vi "RT_PCC_Control_v02b_clean.vi"() -> ()   [LabVIEW 2015]
uses:
  subVIs/PCC case typedef.ctl
  subVIs/Data_Queue_Command.ctl
  <vilib>/Platform/TimedLoop/XDataNode/timing_clust.ctl
  <vilib>/Platform/TimedLoop/XDataNode/nitl_modes.ctl
  <vilib>/Platform/TimedLoop/XDataNode/wakeup.ctl
  <vilib>/FPGAPlugInAG/cRIO-9068/niLvFpga_Open_cRIO-9068.vi
  <vilib>/rvi/interface/common/dynamic/niFpgaDynamicAddResources.vi
  <vilib>/Utility/error.llb/Error Cluster From Error Code.vi
  <vilib>/rvi/errors/niLvFpgaAdjustHostInterfaceError.vi
  <vilib>/FPGAPlugInAG/Dynamic/niLvFpga_Close_Dynamic.vi
  <vilib>/Modbus/slave/Create Slave Instance (TCP).vi
  <vilib>/Platform/TimedLoop/XDataNode/XDataNode.xnode
  <vilib>/rvi/interface/nirviOpenFPGA/nirviOpenFPGA.xnode
  FPGA Bitfiles/RTDSPCCControl_FPGA_RTDS_PCC_v02b_clean.lvbitx
  <vilib>/rvi/interface/nirviReadWriteControl/nirviReadWriteControl.xnode
  <vilib>/rvi/interface/nirviCloseFPGA/nirviCloseFPGA.xnode
  <vilib>/Modbus/slave/Modbus Slave.lvclass
  NiFpgaLv.dll
  <vilib>/rvi/interface/Simulation/niFpgaSimulationCallBeginRW.vi
  2015 SP1 Support Files/Project Dependencies/Common/Modbus Data Conversion.llb/Modbus Data Conversion.lvlib
  <vilib>/Platform/TimedLoop/XDataNode/XDNodeRunTimeDep.lvlib
panel:
  out "Paused?":bool
  in  "unpause":bool
  out "Enable Resync":bool
  out "Graph Data":sgl[][](graph)
  out "state machine loop time":u32
  out "PLL Time MG":u32
  in  "RMS reset":bool
  out "Grid Voltage":sgl[][](graph)
  out "Current":sgl[][](graph)
  out "Grid Freq":sgl[][](graph)
  in  "LPF enable":bool=TRUE
  out "RMS Time":u32
  out "Resync Time":u32
  out "S, P, & Q":cluster{sgl, sgl, sgl}(graph)
  in  "Use Angle for Q":bool
  out "error out":errorcluster
  out "RMS Computation Valid":bool
  out "Comm\nTimeout":bool
  out "V&I Cluster":cluster{sgl, sgl, sgl, sgl, sgl, sgl}
  out "P Cluster":cluster{sgl, sgl, sgl}
  out "S Cluster":cluster{sgl, sgl, sgl}
  out "Q Cluster":cluster{sgl, sgl, sgl}
  out "Q Total":sgl
  out "P Total":sgl
  out "S Total":sgl
  in  "Pause":bool
  out "Modbus Values":T1
  out "comm\nstopped":bool
  in  "Input Cluster":T1
  in  "Enable Switching":bool=TRUE
  out "Current state":T2
  in  "stop":bool
  out "Loop rate":u32=1332
  in  "Reset PLL":bool
  out "Open Switch":bool
  out "Close Switch":bool
  out "Switch Closed?":bool
  out "Activate Command":bool
  out "Deactivate Command":bool
  out "Activation Status":bool
  out "Deactivation Status":bool=TRUE
  out "TCP \nConnection Count":u32
  in  "Input register\naddresses":T3={"Ia RMS"=30030, "Ib RMS"=30040, "Ic RMS"=30050, "Vab RMS"=30130, "Vbc RMS"=30140, "Vca RMS"=30150, "Pa"=30230, "Pb"=30240, "Pc"=30250, "Qa"=30330, "Qb"=30340, "Qc"=30350}
  in  "Tab Control":enum32{"Resynchronization", "Normal Operation"}(tab)
  out "V RMS Resync":cluster{dbl, dbl}(graph)
  out "Freq Resync":cluster{dbl, dbl}(graph)
  out "Phase Resync":cluster{dbl, dbl, dbl, dbl}(graph)
  out "V rms":cluster{sgl, sgl}(graph)
  # "IF Error 1 < Limit 1\nOR \n(Error 2 > Limit 2 AND Error 2 < Limit 1)\nTHEN\nResync"
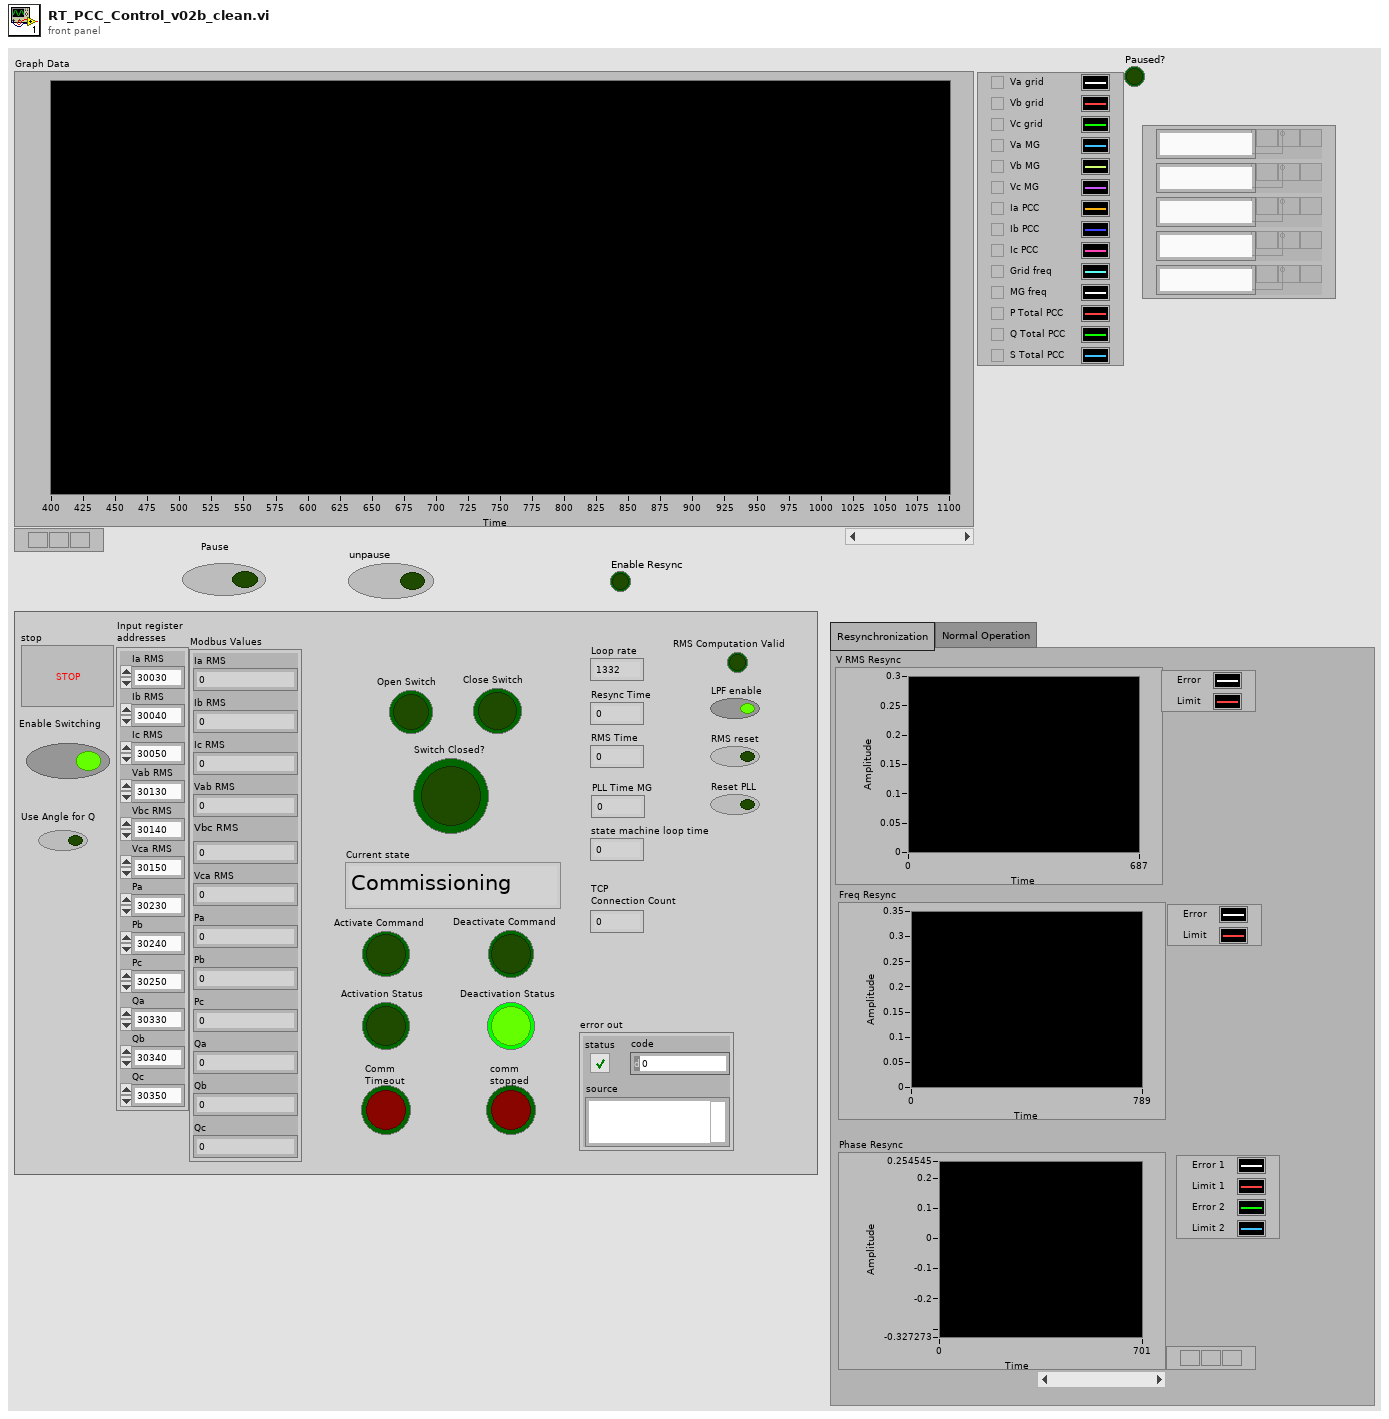
[diagram p1: front panel]
types:
  T1 = cluster{"Ia RMS":sgl, "Ib RMS":sgl, "Ic RMS":sgl, "Vab RMS":sgl, "Vbc RMS":sgl, "Vca RMS":sgl, "Pa":sgl, "Pb":sgl, "Pc":sgl, "Qa":sgl, "Qb":sgl, "Qc":sgl}
  T2 = typedef "PCC case typedef.ctl" = enum16{"Commissioning", "Open", "Synchronize check", "Synchronize", "Closed", "Island watch"}
  T3 = cluster{"Ia RMS":u16, "Ib RMS":u16, "Ic RMS":u16, "Vab RMS":u16, "Vbc RMS":u16, "Vca RMS":u16, "Pa":u16, "Pb":u16, "Pc":u16, "Qa":u16, "Qb":u16, "Qc":u16}
  T4 = typedef "Data_Queue_Command.ctl" = enum16{"Initialize", "Write Sample", "Pull Array", "Close"}
  T5 = typedef "XDNodeRunTimeDep.lvlib/timing_clust.ctl" = cluster{"Expected End [f-1]":u64, "Actual End [f-1]":u64, "Finished Late? [f-1]":bool, "Expected End [i-1]":u64, "Actual End [i-1]":u64, "Finished Late? [i-1]":bool, "Expected Start [i]":u64, "Actual Start [i]":u64, "Expected Start [f]":u64, "Actual Start [f]":u64, "Source Name":string, "Structure Name":string, "Period":i64, "Deadline":i64, "Offset":i64, "Start":i64, "Priority":i32, "Timeout":i32, "Mode":T6, "Wakeup Reason":T7, "Error":errorcluster, "Source Type":string, "Secondary Source Type":string, "Global End Time":u64, "Global Start Time":u64, "Frame Duration":u64, "Iteration Duration":u64, "Assigned CPU":i32, "I/O Scan Engine Mode":u32}
  T6 = typedef "XDNodeRunTimeDep.lvlib/nitl_modes.ctl" = enum32{"No Change", "Process missed periods, maintain original phase", "Discard missed periods, maintain original phase", "Process missed periods, ignore original phase", "Discard missed periods, ignore original phase"}
  T7 = typedef "XDNodeRunTimeDep.lvlib/wakeup.ctl" = enum32{"Normal", "Aborted", "Asynchronous wakeup", "Timing source error", "Timed loop error", "Timeout"}
  T8 = cluster{"Qa":fxp<+/-,46,10>, "Qb":fxp<+/-,46,10>, "Qc":fxp<+/-,46,10>}
  T9 = cluster{"Pa":fxp<+/-,32,10>, "Pb":fxp<+/-,32,10>, "Pc":fxp<+/-,32,10>}
  T10 = cluster{"Vab grid RMS":fxp<+,16,5>, "Vbc grid RMS":fxp<+,16,5>, "Vca grid RMS":fxp<+,16,5>, "Ia RMS":fxp<+,16,5>, "Ib RMS":fxp<+,16,5>, "Ic RMS":fxp<+,16,5>}
  T11 = cluster{"Vab grid RMS":sgl, "Vbc grid RMS":sgl, "Vca grid RMS":sgl, "Ia RMS":sgl, "Ib RMS":sgl, "Ic RMS":sgl}
  T12 = cluster{"Ia":fxp<+/-,24,5>, "Ib":fxp<+/-,24,5>, "Ic":fxp<+/-,24,5>}
  T13 = cluster{"Va":fxp<+/-,18,4>, "Vb":fxp<+/-,18,4>, "Vc":fxp<+/-,18,4>}
  T14 = cluster{"Va grid":sgl, "Vb grid":sgl, "Vc grid":sgl, "Ia":sgl, "Ib":sgl, "Ic":sgl}
  T15 = cluster{"Ia RMS":fxp<+,16,5>, "Ib RMS":fxp<+,16,5>, "Ic RMS":fxp<+,16,5>, "Vab grid RMS":fxp<+,16,5>, "Vbc grid RMS":fxp<+,16,5>, "Vca grid RMS":fxp<+,16,5>}
  T16 = cluster{"Ia RMS":sgl, "Ib RMS":sgl, "Ic RMS":sgl, "Vab grid RMS":sgl, "Vbc grid RMS":sgl, "Vca grid RMS":sgl}
  T17 = cluster{"Freq error":fxp<+,32,8>, "Freq constant":fxp<+,32,8>}
  T18 = cluster{"Phase angle error":fxp<+,32,1>, "Phase angle constant":fxp<+,32,1>, fxp<+/-,33,2>, "y":fxp<+,32,1>}
  T19 = cluster{fxp<+,27,5>, "Vgrid RMS constant (off grid)":fxp<+,27,5>}
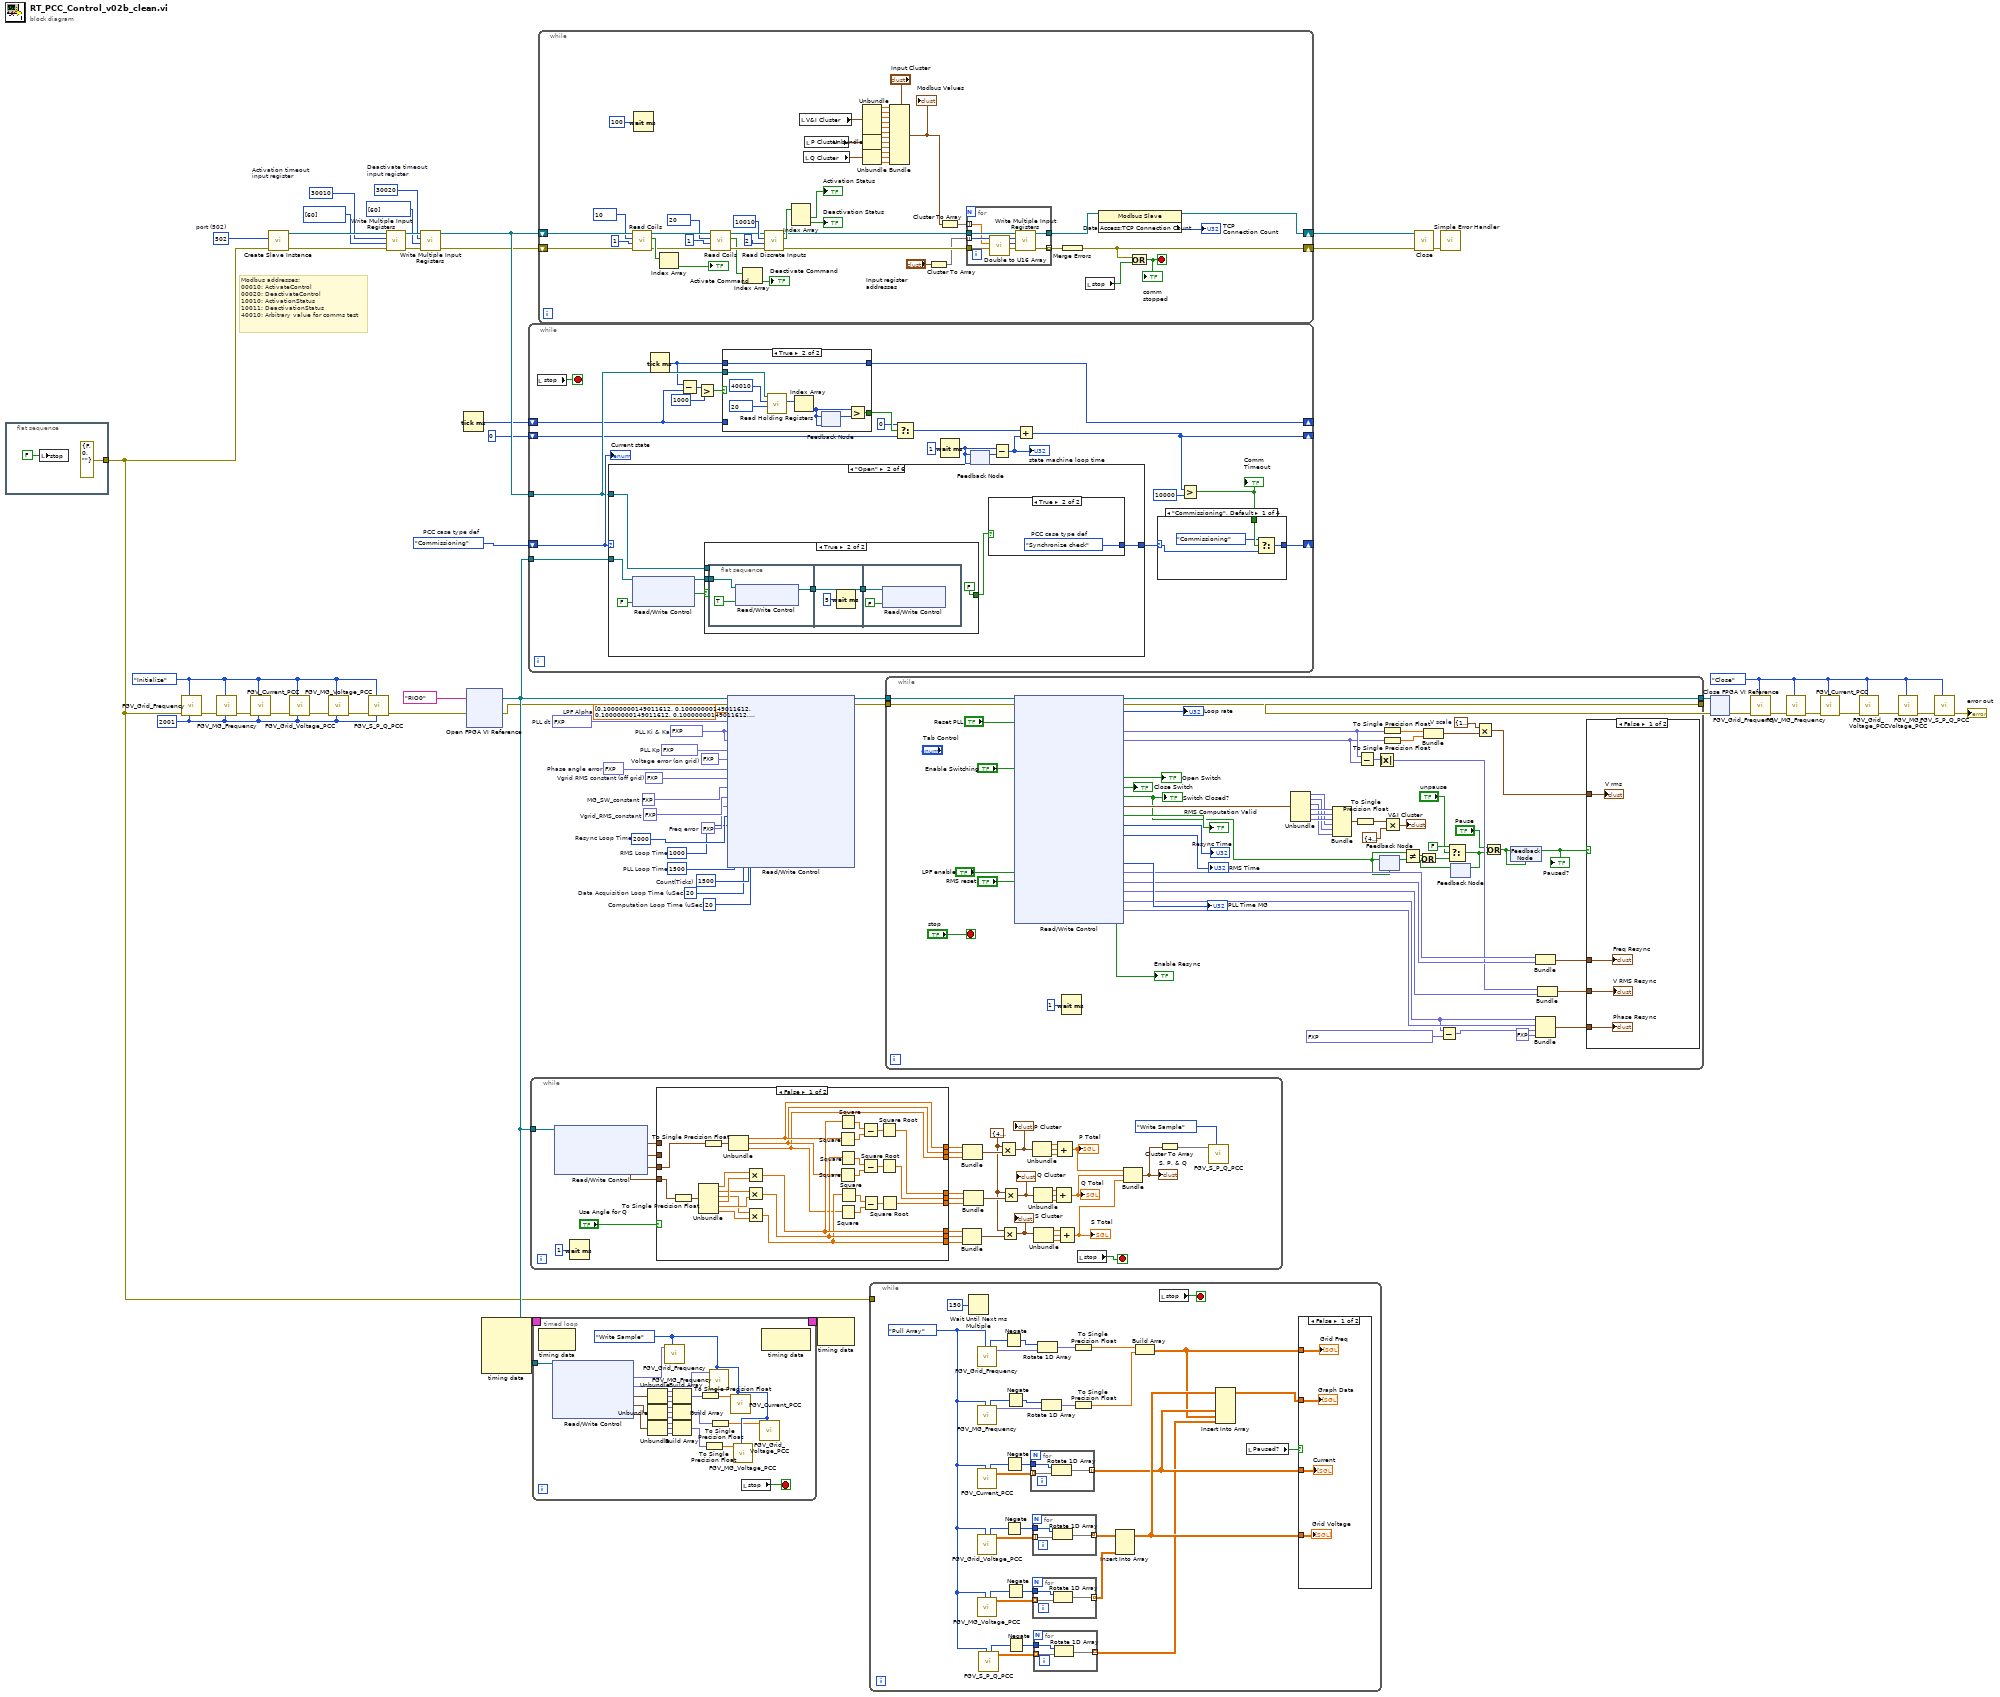
[diagram p0: block diagram]
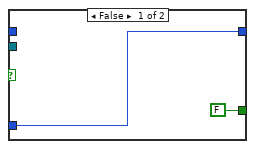
[diagram p2: hidden frame]
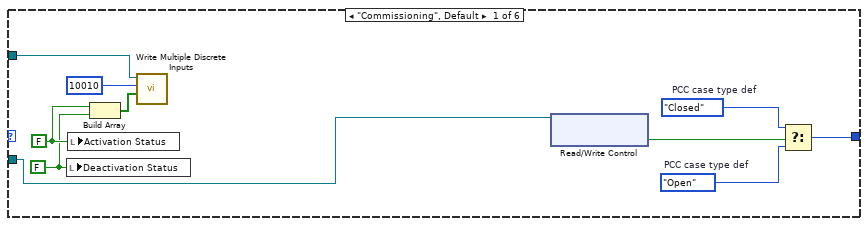
[diagram p6: hidden frame]
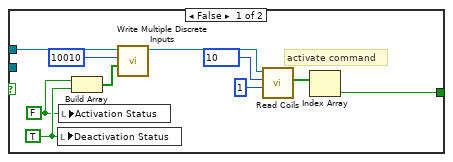
[diagram p7: hidden frame]
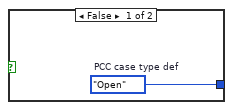
[diagram p8: hidden frame]
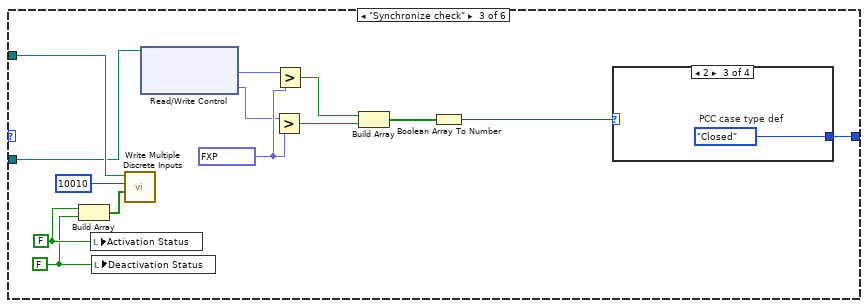
[diagram p9: hidden frame]
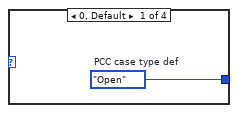
[diagram p10: hidden frame]
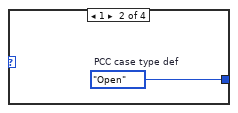
[diagram p11: hidden frame]
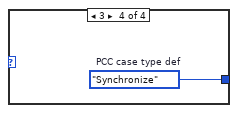
[diagram p12: hidden frame]
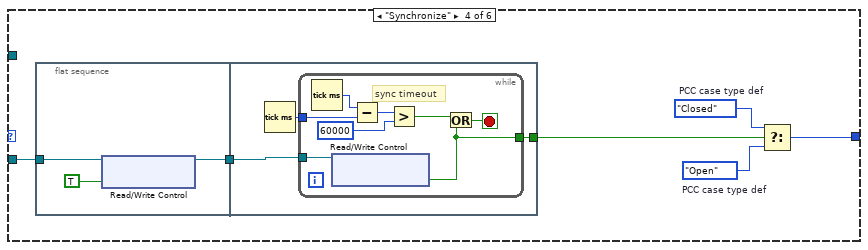
[diagram p13: hidden frame]
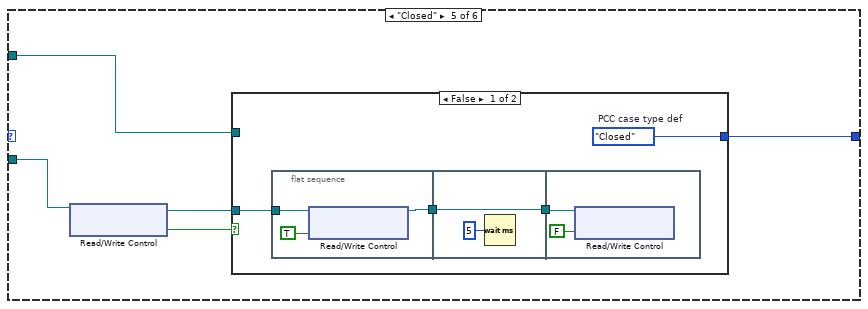
[diagram p14: hidden frame]
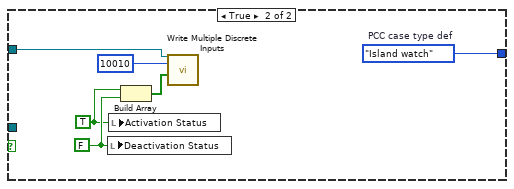
[diagram p15: hidden frame]
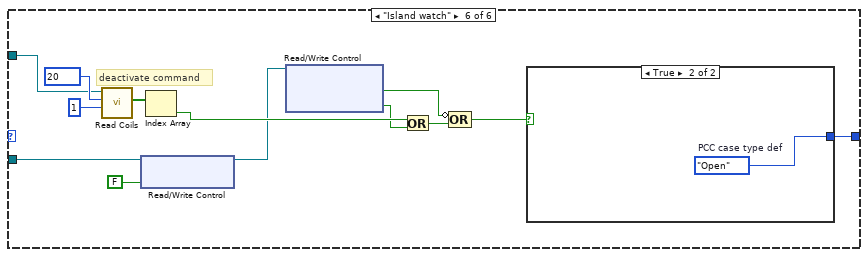
[diagram p16: hidden frame]
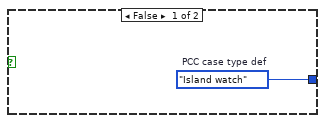
[diagram p17: hidden frame]
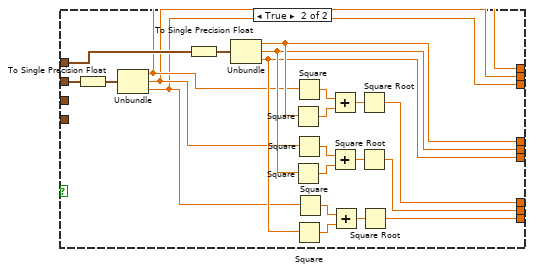
[diagram p19: hidden frame]
diagram:
  w56 = u16 502  # port (502)
  w9 = u32 20  # Computation Loop Time (uSec)
  w10 = u32 20  # Data Acquisition Loop Time (uSec)
  w11 = u32 1000  # RMS Loop Time
  w12 = u32 2000  # Resync Loop Time
  w13 = fxp<+,32,8> 0.30000001192092896  # Freq error
  w14 = fxp<+,27,9> 2.700000762939453  # Vgrid_RMS_constant
  w15 = fxp<+/-,24,5> 4.0  # MG_SW_constant
  w16 = fxp<+,27,5> 0.26999998092651367  # Vgrid RMS constant (off grid)
  w17 = fxp<+,32,1> 0.05599999986588955  # Phase angle error
  w18 = fxp<+/-,28,7> 0.26999998092651367  # Voltage error (on grid)
  w19 = u32 1500  # PLL Loop Time
  w20 = fxp<+,16,6> 0.0126953125  # PLL Kp
  w21 = fxp<+,16,9> 0.1015625  # PLL Ki & Ka
  w22 = fxp<+,24,-5> 3.750063478946686e-05  # PLL dt
  w23 = u32 1500  # Count(Ticks)
  w24 = sgl[] [0.1, 0.1, 0.1, 0.1, 0.1, 0.1, 0.1, 0.1, 0.1]  # LPF Alpha
  w33 = PCC_case_typedef."Commissioning"  # PCC case type def
  w2 = Data_Queue_Command."Close" ("Command")
  w6 = Data_Queue_Command."Initialize" ("Command")
  w5 = 2001 ("Buffer Size")
  w45 = u16 30020  # Deactivate timeout input register
  w47 = u16 30010  # Activation timeout input register
  # "Modbus addresses:\n00010: ActivateControl\n00020: DeactivateControl\n10010: ActivationStatus\n10011: DeactivationStatus\n40010: Arbitrary value for comms test"
  n1 = flat-sequence {
    tunnel: [errorcluster {"status"=FALSE, "code"=0, "source"=""} ("error constant")] -> w1
    frame #0 {
      n2 = local write "stop"(FALSE ("stop")) -> ()
    }
  }
  n3 = call "FGV_Grid_Frequency.vi"("Buffer Size"=w5, "Command"=w6, "error in (no error)"=w1) -> ("error out"=w39:errorcluster)  [unwired: 6 in, 2 out]
  n4 = call "FGV_MG_Frequency.vi"("Buffer Size"=w5, "Command"=w6, "error in (no error)"=w39) -> ("error out"=w40:errorcluster)  [unwired: 6 in, 2 out]
  n5 = call "FGV_Current_PCC.vi"("Buffer Size"=w5, "Command"=w6, "error in (no error)"=w40) -> ("error out"=w42:errorcluster)  [unwired: 6 in, 2 out]
  n6 = call-poly <vilib>:"Create Slave Instance.vi"("error in (no error)"=w1, "port (502)"=w56) -> ("error out"=w52:errorcluster, "TCP slave instance"=w50:refnum<class "Modbus Slave.lvclass">)  [unwired: 8 in]
  n7 = call "FGV_Grid_Voltage_PCC.vi"("Buffer Size"=w5, "Command"=w6, "error in (no error)"=w42) -> ("error out"=w41:errorcluster)  [unwired: 6 in, 2 out]
  n8 = call "FGV_MG_Voltage_PCC.vi"("Buffer Size"=w5, "Command"=w6, "error in (no error)"=w41) -> ("error out"=w8:errorcluster)  [unwired: 6 in, 2 out]
  n9 = call "FGV_S_P_Q_PCC.vi"("Buffer Size"=w5, "Command"=w6, "error in (no error)"=w8) -> ("error out"=w7:errorcluster)  [unwired: 6 in, 2 out]
  n10 = call-dynamic "Write Multiple Input Registers.vi"("error in (no error)"=w52, "input register values"=u16[] [60], "starting address"=w47, "Modbus slave in"=w50) -> ("error out"=w53:errorcluster, "Modbus slave out"=w51:refnum<class "Modbus Slave.lvclass">)  [unwired: 6 in]
  n11 = call-dynamic "Write Multiple Input Registers.vi"("error in (no error)"=w53, "input register values"=u16[] [60], "starting address"=w45, "Modbus slave in"=w51) -> ("error out"=w43:errorcluster, "Modbus slave out"=w49:refnum<class "Modbus Slave.lvclass">)  [unwired: 6 in]
  n12 = Tick Count (ms)() -> (millisecond timer value=w31:u32)
  n13 = xnode "Open FPGA VI Reference"("error in"=w7, "resource name"=tag "RIO0") -> ("FPGA VI Reference Out"=w28:refnum<k20>, "error out"=w26:errorcluster)
  n14 = node-c288() -> (w30:T5)  [unwired: 4 in]
  n15 = while {
    shift-right: [w78] -> _
    shift-left: w33 -> [w84]
    tunnel: w49 -> [w81]
    tunnel: w28 -> [w83]
    shift-right: [w79] -> _
    shift-left: u16 0 ("element") -> [w80]
    shift-right: [w76] -> _
    shift-left: w31 -> [w77]
    stop <- w82 stop-if-true
    n16 = local read "stop"() -> (w82:bool)
    n17 = case shown="\"Open\"" w84 {
      tunnel: [w106 w118 w153 w165 w183 w213] -> w71
      tunnel: w81 -> [w111 w117 w145 _ w184 w209]
      tunnel: w83 -> [w102 w115 w144 w163 w181 w203]
      frame "Commissioning", Default {
        w104 = PCC_case_typedef."Open"  # PCC case type def
        w108 = FALSE ("Open switch")
        w107 = FALSE ("Open switch")
        w105 = PCC_case_typedef."Closed"  # PCC case type def
        n18 = local write "Deactivation Status"(w107) -> ()
        n19 = local write "Activation Status"(w108) -> ()
        n20 = Build Array(w108, w107) -> (w109:bool[])
        n21 = call-dynamic "Write Multiple Discrete Inputs.vi"("discrete input values"=w109, "starting address"=u16 10010, "Modbus slave in"=w111) -> ()  [unwired: 7 in, 2 out]
        n22 = xnode "Read/Write Control"("FPGA VI Reference In"=w102) -> ("Switch Closed?"=w103:bool)  [unwired: 1 in, 2 out]
        n23 = Select(t=w105, s=w103, f=w104) -> (s? t:f=w106:T2)
      }
      frame "Open" {
        n24 = xnode "Read/Write Control"("FPGA VI Reference In"=w115, "Enable Resync"=FALSE) -> ("FPGA VI Reference Out"=w113:refnum<k20>, "Switch Closed?"=w114:bool)  [unwired: 1 in, 1 out]
        n25 = case shown="True" w114 {
          tunnel: w117 -> [w124 _]
          tunnel: [w119 FALSE ("Boolean")] -> w116
          tunnel: w113 -> [_ w132]
          frame False {
            w127 = FALSE ("Deactivate status")
            w128 = TRUE ("Deactivate status")
            # "activate command"
            n26 = local write "Deactivation Status"(w128) -> ()
            n27 = local write "Activation Status"(w127) -> ()
            n28 = Build Array(w127, w128) -> (w126:bool[])
            n29 = call-dynamic "Write Multiple Discrete Inputs.vi"("discrete input values"=w126, "starting address"=u16 10010, "Modbus slave in"=w124) -> ("Modbus slave out"=w120:refnum<class "Modbus Slave.lvclass">)  [unwired: 7 in, 1 out]
            n30 = call-dynamic "Read Coils.vi"("number of coils"=u16 1, "starting address"=u16 10, "Modbus slave in"=w120) -> ("coil values"=w123:bool[])  [unwired: 6 in, 2 out]
            n31 = Index Array(array=w123) -> (element=w119:bool)  [unwired: 1 in]
          }
          frame True {
            n32 = flat-sequence {
              tunnel: w132 -> [w135]
              tunnel: [w133] -> w131
              tunnel: w131 -> [w136]
              tunnel: [w136] -> w130
              tunnel: w130 -> [w138]
              frame #0 {
                n33 = xnode "Read/Write Control"("FPGA VI Reference In"=w135, "Manually Open"=TRUE) -> ("FPGA VI Reference Out"=w133:refnum<k20>)  [unwired: 1 in, 1 out]
              }
              frame #1 {
                n34 = Wait (ms)(milliseconds to wait=u32 5) -> ()  [unwired: 1 out]
              }
              frame #2 {
                n35 = xnode "Read/Write Control"("FPGA VI Reference In"=w138, "Manually Open"=FALSE) -> ()  [unwired: 1 in, 2 out]
              }
            }
          }
        }
        n36 = case shown="True" w116 {
          tunnel: [w140 w141] -> w118
          frame False {
            w140 = PCC_case_typedef."Open"  # PCC case type def
          }
          frame True {
            w141 = PCC_case_typedef."Synchronize check"  # PCC case type def
          }
        }
      }
      frame "Synchronize check" {
        w147 = FALSE ("Deactivate status")
        w146 = FALSE ("Deactivate status")
        w150 = fxp<+,5,-3> 0.1015625 ("y")
        n37 = Build Array(w147, w146) -> (w148:bool[])
        n38 = local write "Activation Status"(w147) -> ()
        n39 = local write "Deactivation Status"(w146) -> ()
        n40 = call-dynamic "Write Multiple Discrete Inputs.vi"("discrete input values"=w148, "starting address"=u16 10010, "Modbus slave in"=w145) -> ()  [unwired: 7 in, 2 out]
        n41 = xnode "Read/Write Control"("FPGA VI Reference In"=w144) -> ("Microgrid RMS"=w143:fxp<+,27,5>, "Grid RMS"=w142:fxp<+,27,5>)  [unwired: 1 in, 2 out]
        n42 = Greater?(x=w142, y=w150) -> (0:w151:bool)
        n43 = Greater?(x=w143, y=w150) -> (0:w152:bool)
        n44 = Build Array(w152, w151) -> (w155:bool[])
        n45 = Boolean Array To Number(Boolean array=w155) -> (number=w154:u32)
        n46 = case shown="2" w154 {
          tunnel: [w156 w157 w158 w159] -> w153
          frame 0, Default {
            w156 = PCC_case_typedef."Open"  # PCC case type def
          }
          frame 1 {
            w157 = PCC_case_typedef."Open"  # PCC case type def
          }
          frame 2 {
            w158 = PCC_case_typedef."Closed"  # PCC case type def
          }
          frame 3 {
            w159 = PCC_case_typedef."Synchronize"  # PCC case type def
          }
        }
      }
      frame "Synchronize" {
        w164 = PCC_case_typedef."Closed"  # PCC case type def
        w160 = PCC_case_typedef."Open"  # PCC case type def
        n47 = flat-sequence {
          tunnel: w163 -> [w168]
          tunnel: [w167] -> w162
          tunnel: w162 -> [w170]
          tunnel: [w169] -> w161
          frame #0 {
            n48 = xnode "Read/Write Control"("FPGA VI Reference In"=w168, "Enable Resync"=TRUE) -> ("FPGA VI Reference Out"=w167:refnum<k20>)  [unwired: 1 in, 1 out]
          }
          frame #1 {
            n49 = Tick Count (ms)() -> (millisecond timer value=w171:u32)
            n50 = while {
              tunnel: w171 -> [w178]
              tunnel: w170 -> [w174]
              tunnel: [w172] -> w169
              stop <- w175 stop-if-true
              # "sync timeout"
              n51 = Tick Count (ms)() -> (millisecond timer value=w179:u32)
              n52 = xnode "Read/Write Control"("FPGA VI Reference In"=w174) -> ("Switch Closed?"=w172:bool)  [unwired: 1 in, 2 out]
              n53 = Subtract(x=w179, y=w178) -> (x-y=w177:u32)
              n54 = Greater?(x=w177, y=u32 60000) -> (0:w173:bool)
              n55 = Or(x=w173, y=w172) -> (x .or. y?=w175:bool)
            }
          }
        }
        n56 = Select(t=w164, s=w161, f=w160) -> (s? t:f=w165:T2)
      }
      frame "Closed" {
        n57 = xnode "Read/Write Control"("FPGA VI Reference In"=w181) -> ("FPGA VI Reference Out"=w180:refnum<k20>, "Switch Closed?"=w182:bool)  [unwired: 1 in, 1 out]
        n58 = case shown="False" w182 {
          tunnel: w184 -> [_ w197]
          tunnel: [w188 w196] -> w183
          tunnel: w180 -> [w187 _]
          frame False {
            w188 = PCC_case_typedef."Closed"  # PCC case type def
            n59 = flat-sequence {
              tunnel: w187 -> [w190]
              tunnel: [w189] -> w185
              tunnel: [w192] -> w186
              tunnel: w185 -> [w192]
              tunnel: w186 -> [w195]
              frame #0 {
                n60 = xnode "Read/Write Control"("FPGA VI Reference In"=w190, "Manually Close"=TRUE ("Manually Open")) -> ("FPGA VI Reference Out"=w189:refnum<k20>)  [unwired: 1 in, 1 out]
              }
              frame #1 {
                n61 = Wait (ms)(milliseconds to wait=u32 5) -> ()  [unwired: 1 out]
              }
              frame #2 {
                n62 = xnode "Read/Write Control"("FPGA VI Reference In"=w195, "Manually Close"=FALSE ("Manually Open")) -> ()  [unwired: 1 in, 2 out]
              }
            }
          }
          frame True {
            w196 = PCC_case_typedef."Island watch"  # PCC case type def
            w200 = TRUE ("Deactivate status")
            w201 = FALSE ("Deactivate status")
            n63 = local write "Deactivation Status"(w201) -> ()
            n64 = local write "Activation Status"(w200) -> ()
            n65 = Build Array(w200, w201) -> (w199:bool[])
            n66 = call-dynamic "Write Multiple Discrete Inputs.vi"("discrete input values"=w199, "starting address"=u16 10010, "Modbus slave in"=w197) -> ()  [unwired: 7 in, 2 out]
          }
        }
      }
      frame "Island watch" {
        # "deactivate command"
        n67 = call-dynamic "Read Coils.vi"("number of coils"=u16 1, "starting address"=u16 20, "Modbus slave in"=w209) -> ("coil values"=w210:bool[])  [unwired: 6 in, 2 out]
        n68 = xnode "Read/Write Control"("FPGA VI Reference In"=w203, "Enable Resync"=FALSE) -> ("FPGA VI Reference Out"=w202:refnum<k20>)  [unwired: 1 in, 1 out]
        n69 = Index Array(array=w210) -> (element=w208:bool)  [unwired: 1 in]
        n70 = xnode "Read/Write Control"("FPGA VI Reference In"=w202) -> ("Switch Closed?"=w206:bool, "Open Switch"=w205:bool)  [unwired: 1 in, 2 out]
        n71 = Or(x=w208, y=w205) -> (x .or. y?=w207:bool)
        n72 = Compound Arithmetic op=OR(invert w206, w207) -> (w214:bool)
        n73 = case shown="True" w214 {
          tunnel: [w215 w216] -> w213
          frame False {
            w215 = PCC_case_typedef."Island watch"  # PCC case type def
          }
          frame True {
            w216 = PCC_case_typedef."Open"  # PCC case type def
          }
        }
      }
    }
    n74 = Tick Count (ms)() -> (millisecond timer value=w65:u32)
    n75 = Subtract(x=w65, y=w77) -> (x-y=w68:u32)
    n76 = Greater?(x=w68, y=u32 1000) -> (0:w66:bool)
    n77 = case shown="True" w66 {
      tunnel: w81 -> [_ w87]
      tunnel: [FALSE w89] -> w75
      tunnel: w65 -> [_ w88]
      tunnel: [w85 w88] -> w76
      tunnel: w77 -> [w85 _]
      frame False {
      }
      frame True {
        n78 = call-dynamic "Read Holding Registers.vi"("number of holding registers"=u16 20 ("starting address"), "starting address"=u16 40010, "Modbus slave in"=w87) -> ("register values"=w94:u16[])  [unwired: 6 in, 2 out]
        n79 = Index Array(array=w94) -> (element=w92:u16)  [unwired: 1 in]
        n80 = feedback #1(w92) -> (w93:u16)
        n81 = feedback-in #1(w92) -> ()
        n82 = Greater?(x=w92, y=w93) -> (0:w89:bool)
      }
    }
    n83 = Select(t=u16 0, s=w75, f=w80) -> (s? t:f=w64:u32)
    n84 = Wait (ms)(milliseconds to wait=u32 1) -> (millisecond timer value=w62:u32)
    n85 = feedback #2(w62) -> (w69:u32)
    n86 = feedback-in #2(w62) -> ()
    n87 = Subtract(x=w62, y=w69) -> (x-y=w63:u32)
    "state machine loop time" <- w63
    n88 = Add(x=w64, y=w63) -> (x+y=w79:u32)
    n89 = Greater?(x=w79, y=u16 10000) -> (0:w70:bool)
    "Comm\nTimeout" <- w70
    n90 = case shown="\"Commissioning\", Default" w71 {
      selector: w71 -> [w97 w99 w100 w101]
      tunnel: [w96 w99 w100 w101] -> w78
      tunnel: w70 -> [w98 _ _ _]
      frame "Commissioning", Default {
        n91 = Select(t=PCC_case_typedef."Commissioning", s=w98, f=w97) -> (s? t:f=w96:T2)
      }
      frame "Open" {
      }
      frame "Closed" {
      }
      frame "Island watch" {
      }
    }
    "Current state" <- w84
  }
  n92 = while {
    tunnel: w28 -> [w254]
    stop <- w224 stop-if-true
    w220 = cluster{sgl, sgl, sgl} {4000.0, 4000.0, 4000.0} ("x")
    n93 = xnode "Read/Write Control"("FPGA VI Reference In"=w254) -> ("Reactive Power"=w252:T8, "Real Power (from angle)"=w251:T9, "Real Power (from mean)"=w250:T9, "Analog rms output"=w239:T10)  [unwired: 1 in, 2 out]
    n94 = Wait (ms)(milliseconds to wait=u32 1) -> ()  [unwired: 1 out]
    n95 = case shown="False" "Use Angle for Q" {
      tunnel: w252 -> [_ w302]
      tunnel: w251 -> [_ w304]
      tunnel: w250 -> [w282 _]
      tunnel: w239 -> [w281 _]
      tunnel: [w262 w292] -> w233
      tunnel: [w263 w291] -> w232
      tunnel: [w264 w290] -> w231
      tunnel: [w261 w289] -> w230
      tunnel: [w260 w288] -> w229
      tunnel: [w259 w287] -> w228
      tunnel: [w258 w286] -> w227
      tunnel: [w257 w285] -> w226
      tunnel: [w256 w284] -> w225
      frame False {
        n96 = To Single Precision Float(number=w281) -> (single precision float=w280:T11)
        n97 = Unbundle(w280) -> ("Vab grid RMS"=w279:sgl, "Vbc grid RMS"=w277:sgl, "Vca grid RMS"=w275:sgl, "Ia RMS"=w278:sgl, "Ib RMS"=w276:sgl, "Ic RMS"=w274:sgl)
        n98 = To Single Precision Float(number=w282) -> (single precision float=w283:cluster{"Pa":sgl, "Pb":sgl, "Pc":sgl})
        n99 = Unbundle(w283) -> ("Pa"=w258:sgl, "Pb"=w257:sgl, "Pc"=w256:sgl)
        n100 = Multiply(x=w279, y=w278) -> (x*y=w264:sgl)
        n101 = Multiply(x=w277, y=w276) -> (x*y=w263:sgl)
        n102 = Multiply(x=w275, y=w274) -> (x*y=w262:sgl)
        n103 = Square(x=w258) -> (x^2=w266:sgl)
        n104 = Square(x=w257) -> (x^2=w269:sgl)
        n105 = Square(x=w264) -> (x^2=w267:sgl)
        n106 = Square(x=w263) -> (x^2=w268:sgl)
        n107 = Square(x=w256) -> (x^2=w272:sgl)
        n108 = Square(x=w262) -> (x^2=w273:sgl)
        n109 = Subtract(x=w267, y=w266) -> (x-y=w265:sgl)
        n110 = Subtract(x=w268, y=w269) -> (x-y=w270:sgl)
        n111 = Subtract(x=w273, y=w272) -> (x-y=w271:sgl)
        n112 = Square Root(x=w265) -> (sqrt(x)=w261:sgl)
        n113 = Square Root(x=w270) -> (sqrt(x)=w260:sgl)
        n114 = Square Root(x=w271) -> (sqrt(x)=w259:sgl)
      }
      frame True {
        n115 = To Single Precision Float(number=w304) -> (single precision float=w305:cluster{"Pa":sgl, "Pb":sgl, "Pc":sgl})
        n116 = Unbundle(w305) -> ("Pa"=w286:sgl, "Pb"=w285:sgl, "Pc"=w284:sgl)
        n117 = To Single Precision Float(number=w302) -> (single precision float=w303:cluster{"Qa":sgl, "Qb":sgl, "Qc":sgl})
        n118 = Unbundle(w303) -> ("Qa"=w289:sgl, "Qb"=w288:sgl, "Qc"=w287:sgl)
        n119 = Square(x=w289) -> (x^2=w294:sgl)
        n120 = Square(x=w288) -> (x^2=w297:sgl)
        n121 = Square(x=w286) -> (x^2=w295:sgl)
        n122 = Square(x=w285) -> (x^2=w296:sgl)
        n123 = Square(x=w287) -> (x^2=w300:sgl)
        n124 = Square(x=w284) -> (x^2=w301:sgl)
        n125 = Add(x=w295, y=w294) -> (x+y=w293:sgl)
        n126 = Add(x=w296, y=w297) -> (x+y=w298:sgl)
        n127 = Add(x=w301, y=w300) -> (x+y=w299:sgl)
        n128 = Square Root(x=w293) -> (sqrt(x)=w290:sgl)
        n129 = Square Root(x=w298) -> (sqrt(x)=w291:sgl)
        n130 = Square Root(x=w299) -> (sqrt(x)=w292:sgl)
      }
    }
    n131 = Bundle(w231, w232, w233) -> (w238:cluster{sgl, sgl, sgl})  [unwired: 1 in]
    n132 = Bundle("Pa"=w227, "Pb"=w226, "Pc"=w225) -> (w243:cluster{"Pa":sgl, "Pb":sgl, "Pc":sgl})  [unwired: 1 in]
    n133 = Bundle("Qa"=w230, "Qb"=w229, "Qc"=w228) -> (w245:cluster{"Qa":sgl, "Qb":sgl, "Qc":sgl})  [unwired: 1 in]
    n134 = Multiply(x=w220, y=w243) -> (x*y=w244:cluster{sgl, sgl, sgl})
    "P Cluster" <- w244
    n135 = Multiply(x=w220, y=w238) -> (x*y=w234:cluster{sgl, sgl, sgl})
    "S Cluster" <- w234
    n136 = Multiply(x=w220, y=w245) -> (x*y=w246:cluster{sgl, sgl, sgl})
    "Q Cluster" <- w246
    n137 = Unbundle(w244) -> (w242:sgl, w241:sgl, w240:sgl)
    n138 = Unbundle(w246) -> (w249:sgl, w248:sgl, w247:sgl)
    n139 = Unbundle(w234) -> (w235:sgl, w236:sgl, w237:sgl)
    n140 = Compound Arithmetic op=ADD(w249, w248, w247) -> (w222:sgl)
    "Q Total" <- w222
    n141 = Compound Arithmetic op=ADD(w242, w241, w240) -> (w223:sgl)
    "P Total" <- w223
    n142 = Compound Arithmetic op=ADD(w235, w236, w237) -> (w221:sgl)
    "S Total" <- w221
    n143 = local read "stop"() -> (w224:bool)
    n144 = Bundle(w223, w222, w221) -> (w219:cluster{sgl, sgl, sgl})  [unwired: 1 in]
    "S, P, & Q" <- w219
    n145 = Cluster To Array(cluster=w219) -> (array=w218:sgl[])
    n146 = call "FGV_S_P_Q_PCC.vi"("Command"=Data_Queue_Command."Write Sample", "Vabc"=w218) -> ()  [unwired: 7 in, 3 out]
  }
  n147 = timed-loop {
    tunnel: w28 -> [w328]
    timing: w30 -> [_]
    timing-out: [_] -> w29
    stop <- w306 stop-if-true
    w327 = Data_Queue_Command."Write Sample" ("Command")
    n148 = node-c288() -> ()  [unwired: 1 in, 1 out]
    n149 = xnode "Read/Write Control"("FPGA VI Reference In"=w328) -> ("Grid  Frequency"=w326:fxp<+,32,8>, "Microgrid  frequency"=w325:fxp<+,32,8>, "Grid Iabc"=w324:T12, "Grid Vabc"=w323:T13, "Microgrid Vabc"=w322:T13)  [unwired: 1 in, 2 out]
    n150 = Unbundle(w324) -> ("Ia"=w321:fxp<+/-,24,5>, "Ib"=w320:fxp<+/-,24,5>, "Ic"=w319:fxp<+/-,24,5>)
    n151 = Unbundle(w323) -> ("Va"=w318:fxp<+/-,18,4>, "Vb"=w317:fxp<+/-,18,4>, "Vc"=w316:fxp<+/-,18,4>)
    n152 = Unbundle(w322) -> ("Va"=w315:fxp<+/-,18,4>, "Vb"=w314:fxp<+/-,18,4>, "Vc"=w313:fxp<+/-,18,4>)
    n153 = call "FGV_Grid_Frequency.vi"("Command"=w327, "Sample"=w326) -> ()  [unwired: 7 in, 3 out]
    n154 = Build Array(w321, w320, w319) -> (w312:fxp<+/-,24,5>[])
    n155 = Build Array(w318, w317, w316) -> (w311:fxp<+/-,18,4>[])
    n156 = Build Array(w315, w314, w313) -> (w310:fxp<+/-,18,4>[])
    n157 = To Single Precision Float(number=w312) -> (single precision float=w309:sgl[])
    n158 = To Single Precision Float(number=w310) -> (single precision float=w307:sgl[])
    n159 = call "FGV_MG_Frequency.vi"("Command"=w327, "Sample"=w325) -> ()  [unwired: 7 in, 3 out]
    n160 = To Single Precision Float(number=w311) -> (single precision float=w308:sgl[])
    n161 = call "FGV_Current_PCC.vi"("Command"=w327, "Iabc"=w309) -> ()  [unwired: 7 in, 3 out]
    n162 = call "FGV_MG_Voltage_PCC.vi"("Command"=w327, "Vabc"=w307) -> ()  [unwired: 7 in, 3 out]
    n163 = local read "stop"() -> (w306:bool)
    n164 = call "FGV_Grid_Voltage_PCC.vi"("Command"=w327, "Vabc"=w308) -> ()  [unwired: 7 in, 3 out]
    n165 = node-c288() -> ()  [unwired: 1 in, 1 out]
  }
  n166 = while {
    shift-right: [w359] -> w58
    shift-left: w49 -> [w375]
    shift-right: [w333] -> w57
    shift-left: w43 -> [w374]
    stop <- w378 stop-if-true
    n167 = call-dynamic "Read Coils.vi"("error in (no error)"=w374, "number of coils"=u16 1, "starting address"=u16 10, "Modbus slave in"=w375) -> ("error out"=w367:errorcluster, "coil values"=w379:bool[], "Modbus slave out"=w364:refnum<class "Modbus Slave.lvclass">)  [unwired: 5 in]
    n168 = Wait (ms)(milliseconds to wait=u32 100) -> ()  [unwired: 1 out]
    n169 = Index Array(array=w379) -> (element=→"Activate Command":bool)  [unwired: 1 in]
    n170 = call-dynamic "Read Coils.vi"("error in (no error)"=w367, "number of coils"=u16 1, "starting address"=u16 20, "Modbus slave in"=w364) -> ("error out"=w366:errorcluster, "coil values"=w361:bool[], "Modbus slave out"=w365:refnum<class "Modbus Slave.lvclass">)  [unwired: 5 in]
    n171 = Index Array(array=w361) -> (element=→"Deactivate Command":bool)  [unwired: 1 in]
    n172 = call-dynamic "Read Discrete Inputs.vi"("error in (no error)"=w366, "number of discrete inputs"=u16 2 ("number of coils"), "starting address"=u16 10010 ("address"), "Modbus slave in"=w365) -> ("error out"=w357:errorcluster, "discrete input values"=w372:bool[], "Modbus slave out"=w358:refnum<class "Modbus Slave.lvclass">)  [unwired: 5 in]
    n173 = Index Array(array=w372) -> (element #1=→"Activation Status":bool, element #2=→"Deactivation Status":bool)  [unwired: 2 in]
    n174 = local read "V&I Cluster"() -> (w353:cluster{sgl, sgl, sgl, sgl, sgl, sgl})
    n175 = local read "Q Cluster"() -> (w348:cluster{sgl, sgl, sgl})
    n176 = local read "P Cluster"() -> (w352:cluster{sgl, sgl, sgl})
    n177 = Unbundle(w353) -> (w344:sgl, w343:sgl, w342:sgl, w341:sgl, w340:sgl, w339:sgl)
    n178 = Unbundle(w352) -> (w351:sgl, w350:sgl, w349:sgl)
    n179 = Unbundle(w348) -> (w347:sgl, w346:sgl, w345:sgl)
    n180 = Bundle(cluster="Input Cluster", "Ia RMS"=w344, "Ib RMS"=w343, "Ic RMS"=w342, "Vab RMS"=w341, "Vbc RMS"=w340, "Vca RMS"=w339, "Pa"=w351, "Pb"=w350, "Pc"=w349, "Qa"=w347, "Qb"=w346, "Qc"=w345) -> (w334:T1)
    "Modbus Values" <- w334
    n181 = Cluster To Array(cluster="Input register\naddresses") -> (array=w337:u16[])
    n182 = Cluster To Array(cluster=w334) -> (array=w335:sgl[])
    n183 = for {
      tunnel: w358 -> [w386]
      tunnel: w357 -> [w385]
      tunnel: [w383] -> w332
      tunnel: [w382] -> w338 mode=indexing
      tunnel: w337 -> [w381] mode=indexing
      tunnel: w335 -> [w380] mode=indexing
      n184 = call "Double to U16 Array.vi"("Double"=w380) -> ("U16 Array"=w384:u16[])  [unwired: 10 in]
      n185 = call-dynamic "Write Multiple Input Registers.vi"("error in (no error)"=w385, "input register values"=w384, "starting address"=w381, "Modbus slave in"=w386) -> ("error out"=w382:errorcluster, "Modbus slave out"=w383:refnum<class "Modbus Slave.lvclass">)  [unwired: 6 in]
    }
    n186 = Merge Errors(w338) -> (w333:errorcluster)
    n187 = local read "stop"() -> (w355:bool)
    n188 = property class="Modbus Slave"(reference=w332) -> (reference out=w359:refnum<class "Modbus Slave.lvclass">, "Data Access:TCP Connection Count"=→"TCP \nConnection Count":u32)  [unwired: 1 in, 1 out]
    n189 = Compound Arithmetic op=OR(w333, w355) -> (w378:bool)
    "comm\nstopped" <- w378
  }
  n190 = xnode "Read/Write Control"("FPGA VI Reference In"=w28, "error in"=w26, "LPF Alpha"=w24, "PLL dt"=w22, "Ka"=w21, "Ki"=w21, "Kp"=w20, "Voltage constant (on grid)"=w18, "Phase angle constant"=w17, "Vgrid RMS constant (off grid)"=w16, "MG_SW_constant"=w15, "Vgrid RMS constant (on grid)"=w14, "Freq constant"=w13, "Resync Loop Time"=w12, "RMS Loop Time"=w11, "PLL Loop Time"=w19, "Count(Ticks)"=w23, "Data Acquisition Loop Time (uSec)"=w10, "Computation Loop Time (uSec)"=w9) -> ("FPGA VI Reference Out"=w27:refnum<k20>, "error out"=w25:errorcluster)
  n191 = node-c288(w29) -> ()  [unwired: 1 out]
  n192 = while {
    tunnel: w1 -> [_]
    stop <- w419 stop-if-true
    w395 = Data_Queue_Command."Pull Array" ("Command")
    n193 = Wait Until Next ms Multiple(millisecond multiple=u32 150 ("milliseconds to wait")) -> ()  [unwired: 1 out]
    n194 = call "FGV_Grid_Frequency.vi"("Command"=w395) -> ("Buffer"=w405:fxp<+,32,8>[], "Buffer Index"=w418:i32)  [unwired: 8 in, 1 out]
    n195 = call "FGV_MG_Frequency.vi"("Command"=w395) -> ("Buffer"=w406:fxp<+,32,8>[], "Buffer Index"=w408:i32)  [unwired: 8 in, 1 out]
    n196 = call "FGV_Current_PCC.vi"("Command"=w395) -> ("Buffer"=w415:sgl[][], "Buffer Index"=w417:i32)  [unwired: 8 in, 1 out]
    n197 = call "FGV_Grid_Voltage_PCC.vi"("Command"=w395) -> ("Buffer"=w412:sgl[][], "Buffer Index"=w414:i32)  [unwired: 8 in, 1 out]
    n198 = call "FGV_MG_Voltage_PCC.vi"("Command"=w395) -> ("Buffer"=w409:sgl[][], "Buffer Index"=w411:i32)  [unwired: 8 in, 1 out]
    n199 = call "FGV_S_P_Q_PCC.vi"("Command"=w395) -> ("Buffer"=w392:sgl[][], "Buffer Index"=w394:i32)  [unwired: 8 in, 1 out]
    n200 = Negate(x=w418) -> (-x=w404:i32)
    n201 = Negate(x=w414) -> (-x=w413:i32)
    n202 = Negate(x=w417) -> (-x=w416:i32)
    n203 = Negate(x=w408) -> (-x=w407:i32)
    n204 = Negate(x=w411) -> (-x=w410:i32)
    n205 = Negate(x=w394) -> (-x=w393:i32)
    n206 = for {
      tunnel: w416 -> [w435]
      tunnel: w415 -> [w434] mode=indexing
      tunnel: [w433] -> w390 mode=indexing
      n207 = Rotate 1D Array(1:w434, 2:w435) -> (0:w433:sgl[])
    }
    n208 = for {
      tunnel: w413 -> [w430]
      tunnel: w412 -> [w432] mode=indexing
      tunnel: [w431] -> w402 mode=indexing
      n209 = Rotate 1D Array(1:w432, 2:w430) -> (0:w431:sgl[])
    }
    n210 = for {
      tunnel: w410 -> [w429]
      tunnel: w409 -> [w428] mode=indexing
      tunnel: [w427] -> w401 mode=indexing
      n211 = Rotate 1D Array(1:w428, 2:w429) -> (0:w427:sgl[])
    }
    n212 = for {
      tunnel: w393 -> [w422]
      tunnel: w392 -> [w421] mode=indexing
      tunnel: [w420] -> w388 mode=indexing
      n213 = Rotate 1D Array(1:w421, 2:w422) -> (0:w420:sgl[])
    }
    n214 = Rotate 1D Array(1:w405, 2:w404) -> (0:w399:fxp<+,32,8>[])
    n215 = Rotate 1D Array(1:w406, 2:w407) -> (0:w397:fxp<+,32,8>[])
    n216 = To Single Precision Float(number=w399) -> (single precision float=w398:sgl[])
    n217 = To Single Precision Float(number=w397) -> (single precision float=w396:sgl[])
    n218 = Insert Into Array(array=w402, new element=w401) -> (w391:sgl[][])  [unwired: 2 in]
    n219 = Build Array(w398, w396) -> (w389:sgl[][])
    n220 = local read "stop"() -> (w419:bool)
    n221 = Insert Into Array(array=w391, new element #1=w390, new element #2=w389, new element #3=w388) -> (w387:sgl[][])  [unwired: 2 in]
    n222 = local read "Paused?"() -> (w400:bool)
    n223 = case shown="False" w400 {
      tunnel: w390 -> [w426 _]
      tunnel: w391 -> [w425 _]
      tunnel: w389 -> [w424 _]
      tunnel: w387 -> [w423 _]
      frame False {
        "Grid Freq" <- w424
        "Current" <- w426
        "Grid Voltage" <- w425
        "Graph Data" <- w423
      }
      frame True {
      }
    }
  }
  n224 = while {
    tunnel: w27 -> [w495]
    tunnel: w25 -> [w494]
    tunnel: [w476] -> w55
    tunnel: [w493] -> w54
    stop <- "stop" stop-if-true
    w460 = cluster{sgl, sgl} {100.0, 100.0}  # V scale
    n225 = xnode "Read/Write Control"("FPGA VI Reference In"=w495, "error in"=w494, "Reset PLL"="Reset PLL", "Enable Switching"="Enable Switching", "LPF enable"="LPF enable", "RMS reset"="RMS reset") -> ("FPGA VI Reference Out"=w476:refnum<k20>, "error out"=w493:errorcluster, "Loop rate"=→"Loop rate":u32, "Grid RMS"=w459:fxp<+,27,5>, "Microgrid RMS"=w458:fxp<+,27,5>, "Open Switch"=→"Open Switch":bool, "Close Switch"=→"Close Switch":bool, "Switch Closed?"=w436:bool, "Analog rms output"=w477:T10, "RMS Computation Valid"=→"RMS Computation Valid":bool, "Resync Time"=→"Resync Time":u32, "RMS Time"=→"RMS Time":u32, "PLL Time MG"=→"PLL Time MG":u32, "Freq error"=w456:fxp<+,32,8>, "Freq constant"=w455:fxp<+,32,8>, "Vgrid RMS constant (off grid)"=w454:fxp<+,27,5>, "Phase angle error"=w451:fxp<+,32,1>, "Phase angle constant"=w452:fxp<+,32,1>, "Enable Resync"=→"Enable Resync":bool)  [unwired: 2 out]
    "Switch Closed?" <- w436
    n226 = Wait (ms)(milliseconds to wait=u32 1) -> ()  [unwired: 1 out]
    n227 = Unbundle(w477) -> ("Vab grid RMS"=w481:fxp<+,16,5>, "Vbc grid RMS"=w480:fxp<+,16,5>, "Vca grid RMS"=w479:fxp<+,16,5>, "Ia RMS"=w484:fxp<+,16,5>, "Ib RMS"=w483:fxp<+,16,5>, "Ic RMS"=w482:fxp<+,16,5>)
    n228 = Bundle("Ia RMS"=w484, "Ib RMS"=w483, "Ic RMS"=w482, "Vab grid RMS"=w481, "Vbc grid RMS"=w480, "Vca grid RMS"=w479) -> (w478:T15)  [unwired: 1 in]
    n229 = To Single Precision Float(number=w478) -> (single precision float=w486:T16)
    n230 = Subtract(x=w459, y=w458) -> (x-y=w457:fxp<+/-,28,6>)
    n231 = Absolute Value(x=w457) -> (abs(x)=w453:fxp<+,27,5>)
    n232 = feedback-in #3(w436) -> ()
    n233 = feedback #3(w436) -> (w446:bool)
    n234 = To Single Precision Float(number=w459) -> (single precision float=w487:sgl)
    n235 = To Single Precision Float(number=w458) -> (single precision float=w489:sgl)
    n236 = Multiply(x=w486, y=T14 {"Va grid"=40.0, "Vb grid"=40.0, "Vc grid"=40.0, "Ia"=173.2, "Ib"=173.2, "Ic"=173.2}) -> (x*y=→"V&I Cluster":cluster{sgl, sgl, sgl, sgl, sgl, sgl})
    n237 = Not Equal?(x=w436, y=w446) -> (x != y?=w445:bool)
    n238 = Bundle(w487, w489) -> (w461:cluster{sgl, sgl})  [unwired: 1 in]
    n239 = Subtract(x=w451, y=fxp<+,32,1> 1.9999999995343387) -> (x-y=w449:fxp<+/-,33,2>)
    n240 = feedback #4() -> (w441:bool)  [unwired: 1 in]
    n241 = Or(x=w445, y=w441) -> (x .or. y?=w444:bool)
    n242 = Select(t=FALSE, s="unpause", f=w444) -> (s? t:f=w440:bool)
    n243 = feedback-in #4(w440) -> ()
    n244 = Multiply(x=w460, y=w461) -> (x*y=w462:cluster{sgl, sgl})
    n245 = Or(x="Pause", y=w440) -> (x .or. y?=w437:bool)
    n246 = feedback-in #5(w437) -> ()
    n247 = feedback #5(w437) -> (w438:bool)
    "Paused?" <- w438
    n248 = Bundle("Freq error"=w456, "Freq constant"=w455) -> (w467:T17)  [unwired: 1 in]
    n249 = Bundle("Phase angle error"=w451, "Phase angle constant"=w452, w449, "y"=fxp<+,32,1> 0.0) -> (w464:T18)  [unwired: 1 in]
    n250 = Bundle(w453, "Vgrid RMS constant (off grid)"=w454) -> (w466:T19)  [unwired: 1 in]
    n251 = case shown="False" w438 {
      tunnel: w467 -> [w496 _]
      tunnel: w464 -> [w498 _]
      tunnel: w466 -> [w497 _]
      tunnel: w462 -> [w499 _]
      frame False {
        "Freq Resync" <- w496
        "Phase Resync" <- w498
        "V RMS Resync" <- w497
        "V rms" <- w499
      }
      frame True {
      }
    }
  }
  n252 = call-dynamic "Close.vi"("error in (no error)"=w57, "Modbus slave in"=w58) -> ("error out"=w59:errorcluster)  [unwired: 9 in]
  n253 = call <vilib>:"Simple Error Handler.vi"("error in (no error)"=w59) -> ()  [unwired: 4 in, 5 out]
  n254 = xnode "Close FPGA VI Reference"("FPGA VI Reference In"=w55, "error in"=w54) -> ("error out"=w38:errorcluster)
  n255 = call "FGV_Grid_Frequency.vi"("Command"=w2, "error in (no error)"=w38) -> ("error out"=w37:errorcluster)  [unwired: 7 in, 2 out]
  n256 = call "FGV_MG_Frequency.vi"("Command"=w2, "error in (no error)"=w37) -> ("error out"=w36:errorcluster)  [unwired: 7 in, 2 out]
  n257 = call "FGV_Current_PCC.vi"("Command"=w2, "error in (no error)"=w36) -> ("error out"=w35:errorcluster)  [unwired: 7 in, 2 out]
  n258 = call "FGV_Grid_Voltage_PCC.vi"("Command"=w2, "error in (no error)"=w35) -> ("error out"=w34:errorcluster)  [unwired: 7 in, 2 out]
  n259 = call "FGV_MG_Voltage_PCC.vi"("Command"=w2, "error in (no error)"=w34) -> ("error out"=w4:errorcluster)  [unwired: 7 in, 2 out]
  n260 = call "FGV_S_P_Q_PCC.vi"("Command"=w2, "error in (no error)"=w4) -> ("error out"=→"error out":errorcluster)  [unwired: 7 in, 2 out]
